vi "Periodic Tasks.vi"(8 "error in":errorcluster) -> ()   [LabVIEW 2017]
doc: "This VI runs in parallel to other robot code. It can contain as many user-defined periodic loops as you need. These can carry out PID or other sorts of timed response."
uses:
  <vilib>/Rock Robotics/WPI/Utilities/WPI_GetSetVariantRefNum.vi
  Robot Global Data.vi
  <vilib>/Rock Robotics/WPI/ThirdParty/Sensors/ADIS16448 IMU/ADIS16448_IMU.lvlib
panel:
  out "Z Angle":dbl
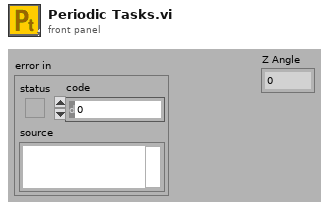
[diagram p1: front panel]
types:
  T1 = typedef "WPI_JoystickDevRef.ctl" = cluster{"Device":T2}
  T2 = typedef "WPI_JoystickDeviceEnum.ctl" = enum16{"USB 0", "USB 1", "USB 2", "USB 3", "USB 4", "USB 5"}
  T3 = typedef "ADIS16448_IMU.lvlib/ADI_IMU_ADIS16448_IMUDevRef.ctl" = cluster{"DevStatus":errorcluster, "Handle":i32, "SPI Bus":T4, "Device Found":bool, "Device Ready":bool, "Yaw Axis":enum16{"X", "Y", "Z"}, "AHRS Algorithm":enum16{"Complementary", "Madgwick"}, "Serial":u16, "Lot ID 2":u16, "Lot ID 1":u16, "Bytes Per Sample":u16, "Calibrate On Open?":bool}
  T4 = typedef "spi_bus.ctl" = enum16{"SPI On-Board, CS0", "SPI On-Board, CS1", "SPI On-Board, CS2", "SPI On-Board, CS3", "SPI MXP", "Invalid"}
  T5 = cluster{"X Angle":dbl, "Y Angle":dbl, "Z Angle":dbl}
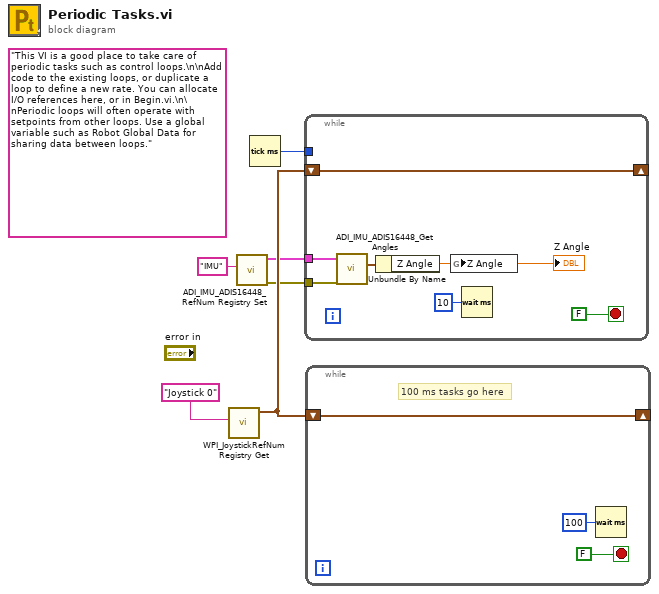
[diagram p0: block diagram]
diagram:
  (unwired) "This VI is a good place to take care of periodic tasks such as control loops.\n\nAdd code to the existing loops, or duplicate a loop to define a new rate. You can allocate I/O references here, or in Begin.vi.\n\nPeriodic loops will often operate with setpoints from other loops. Use a global variable such as Robot Global Data for sharing data between loops."
  n1 = call <vilib>:"WPI_JoystickRefNum Registry Get.vi"("refnum name"="Joystick 0") -> ("JoystickDevRef"=w5:T1)  [unwired: 1 in, 9 out]
  n2 = call <vilib>:"ADI_IMU_ADIS16448_RefNum Registry Set.vi"("refnum name"="IMU") -> ("error out"=w1:errorcluster, "ADI IMU DevRef"=w3:T3)  [unwired: 9 in]
  n3 = Tick Count (ms)() -> (millisecond timer value=w4:u32)
  n4 = while {
    shift-right: [w12] -> _
    shift-left: w5 -> [w12]
    tunnel: w4 -> [_]
    tunnel: w3 -> [w10]
    tunnel: w1 -> [w9]
    stop <- FALSE stop-if-true
    n5 = call <vilib>:"ADI_IMU_ADIS16448_Get Angles.vi"("error in"=w9, "ADI IMU DevRef"=w10) -> ("IMU Angles Out"=w8:T5)  [unwired: 6 in, 3 out]
    n6 = Unbundle By Name(w8) -> ("Z Angle"=w7:dbl)
    "Z Angle" <- w7
    n7 = global write "Robot Global Data.vi" "Z Angle"(w7) -> ()
    n8 = Wait (ms)(milliseconds to wait=u32 10) -> ()  [unwired: 1 out]
  }
  n9 = while {
    shift-right: [w14] -> _
    shift-left: w5 -> [w14]
    stop <- FALSE stop-if-true
    # "100 ms tasks go here"
    n10 = Wait (ms)(milliseconds to wait=u32 100) -> ()  [unwired: 1 out]
  }
